vi "Teleop.vi"(10 "Match Info":T1={"Autonomous Elapsed Seconds"=0.0, "TeleOp Elapsed Seconds"=0.0, "Disabled Elapsed Seconds"=0.0, "Visited Autonomous"=FALSE, "Visited TeleOp"=FALSE, "Visited Disabled"=FALSE, "Autonomous Settings"={"Autonomous Style"=enum."Independent", "VI Refnum"=refnum}}, 11 "Call Context":T2) -> ()   [LabVIEW 2016]
doc: "This VI is called for each TeleOp packet received from the DS where the robot is not disabled. It is often used to read from the joysticks and update I/O or to update setpoints for timed control loops. It should complete and return within 20 milliseconds or it may miss DS packets."
uses:
  <vilib>/Rock Robotics/WPI/DriverStation/WPI_DriverStationDerivedRobotMode.ctl
  <vilib>/Rock Robotics/WPI/DriverStation/WPI_DriverStationMatch Info.ctl
  <vilib>/Rock Robotics/WPI/Utilities/WPI_GetSetVariantRefNum.vi
  <vilib>/Rock Robotics/Network Tables/NT Write Boolean.vi
  <vilib>/Rock Robotics/Network Tables/NT Write Boolean Array.vi
  <vilib>/Rock Robotics/Network Tables/NT Write Numeric Array.vi
  <vilib>/Rock Robotics/WPI/Solenoid/Deprecated/WPI_SolenoidSetBool.vi
  <vilib>/Rock Robotics/WPI/Ultrasonic/WPI_SonarMB1010AnalogRefNum Registry Get.vi
  <vilib>/Rock Robotics/WPI/Ultrasonic/WPI_SonarMB1010AnalogGetRange.vi
  <vilib>/Rock Robotics/Network Tables/NT Read Number.vi
  <vilib>/Rock Robotics/Network Tables/NT Write Number.vi
panel:
  out "gyro":dbl
  out "sonar distance (inches)":dbl
  out "Encoder Loop 2":string
  out "Encoder Loop":dbl
  out "Encoder Rate":dbl
  out "Encoder State":string
  out "Encoder Direction":string
  out "Distance 2":dbl
  out "Angle 2":dbl
  out "Distance":dbl
  out "Enabled":bool
  out "Compressor Running":bool
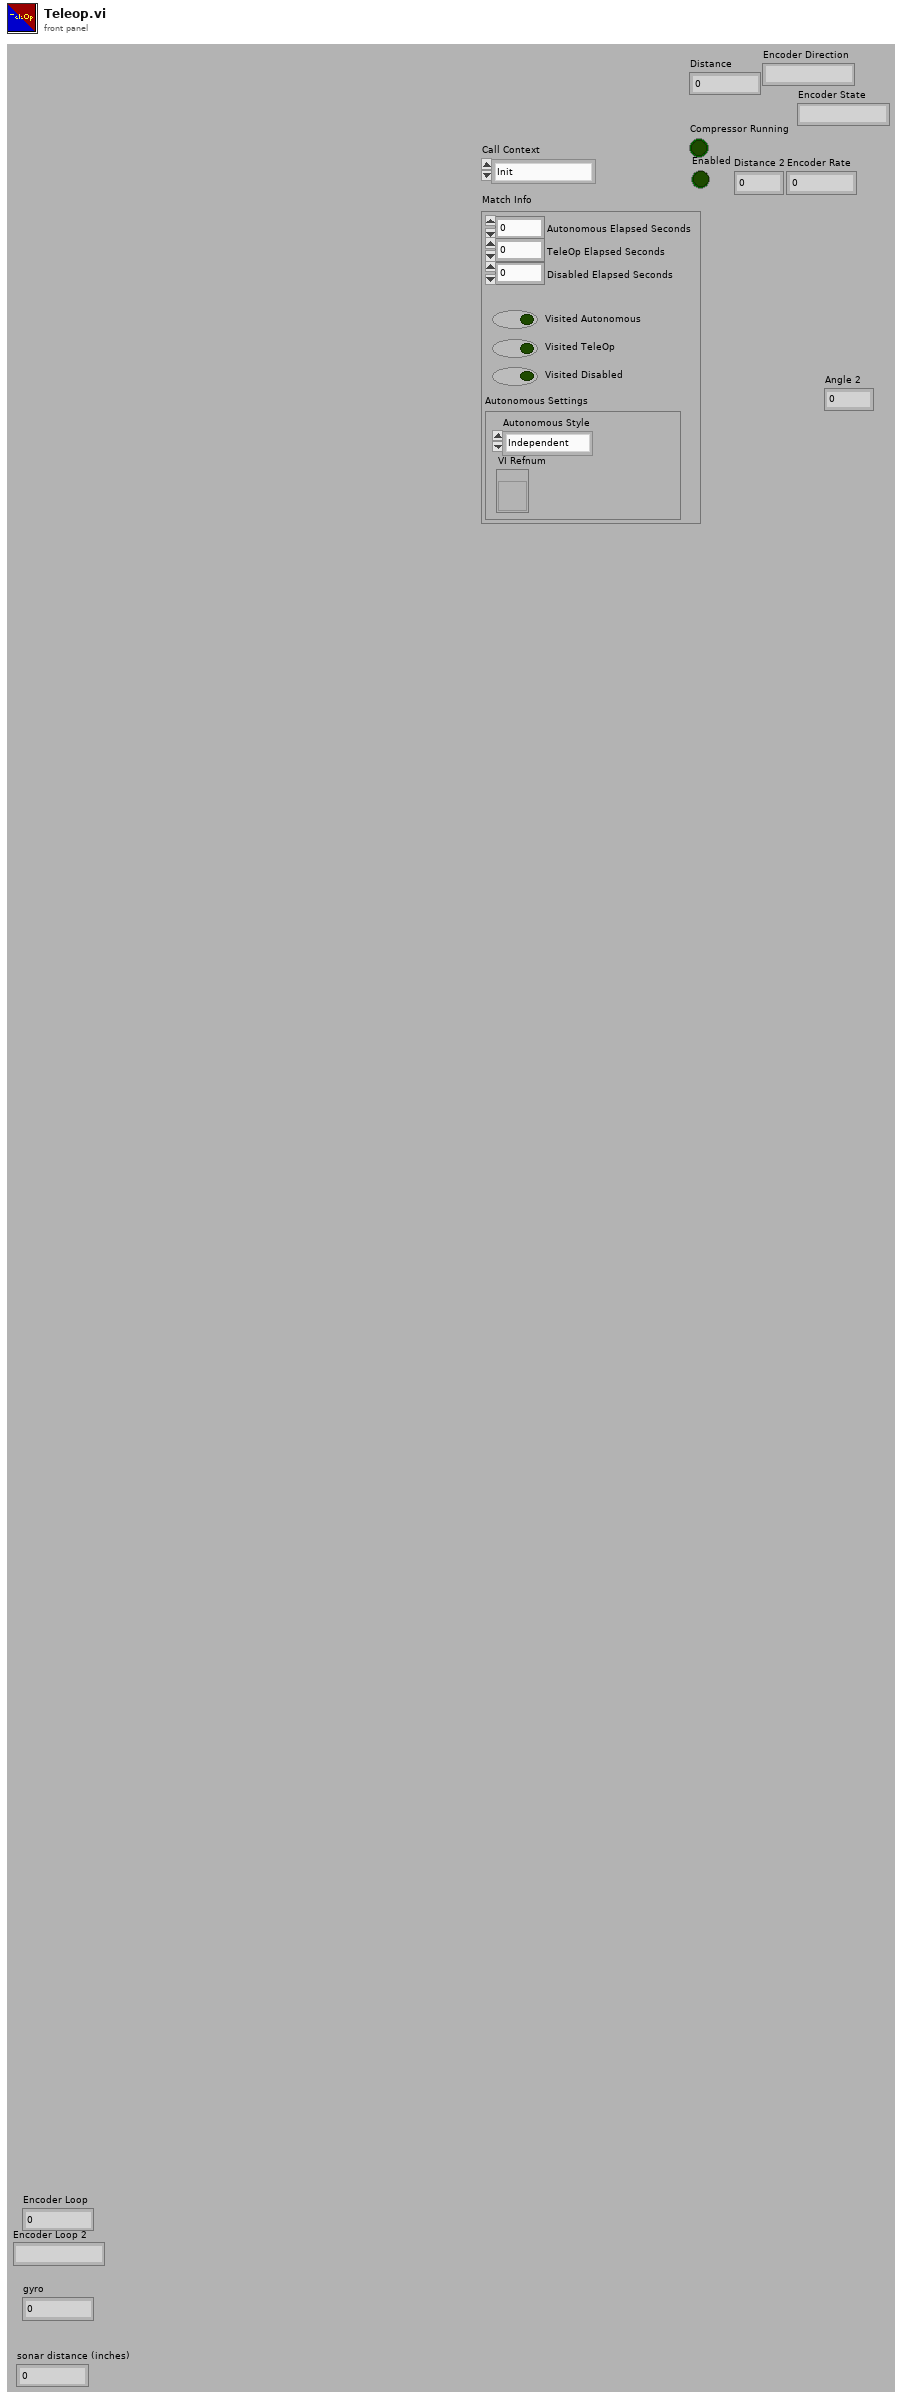
[diagram p1: front panel]
types:
  T1 = typedef "WPI_DriverStationMatch Info.ctl" = cluster{"Autonomous Elapsed Seconds":dbl, "TeleOp Elapsed Seconds":dbl, "Disabled Elapsed Seconds":dbl, "Visited Autonomous":bool, "Visited TeleOp":bool, "Visited Disabled":bool, "Autonomous Settings":cluster{"Autonomous Style":enum16{"Iterative", "Independent"}, "VI Refnum":refnum<vi>}}
  T2 = typedef "WPI_DriverStationDerivedRobotMode.ctl" = enum16{"Init", "Execute", "Stop"}
  T3 = typedef "WPI_EncoderDevRef.ctl" = cluster{"DevStatus":errorcluster, "EncoderIndex":T4, "CounterIndex":T5, "DistancePerCount":dbl, "Decoding Type":T6}
  T4 = typedef "FPGA_EncoderIdx.ctl" = enum8{"Enc 0", "Enc 1", "Enc 2", "Enc 3", "Enc 4", "Enc 5", "Enc 6", "Enc 7", "Invalid"}
  T5 = typedef "FPGA_CounterCtrSystemIndex.ctl" = enum8{"Ctr 0", "Ctr 1", "Ctr 2", "Ctr 3", "Ctr 4", "Ctr 5", "Ctr 6", "Ctr 7", "Invalid"}
  T6 = typedef "WPI_EncoderType.ctl" = enum16{"1x", "2x", "4x"}
  T7 = typedef "WPI_JoystickDevRef.ctl" = cluster{"Device":T8}
  T8 = typedef "WPI_JoystickDeviceEnum.ctl" = enum16{"USB 0", "USB 1", "USB 2", "USB 3", "USB 4", "USB 5"}
  T9 = typedef "WPI_GyroDevRef.ctl" = cluster{"DevStatus":errorcluster, "Analog Channel":T10, "Offset":dbl, "Gain (VoltsPerDegree/Second)":dbl, "Gyro Type":enum16{"Analog", "XRS450"}, "Handle":i32, "SPI Bus":T11, "Device Found":bool, "Sample Rate":dbl, "Calibrate On Open":bool}
  T10 = typedef "FPGA_AIChannel.ctl" = enum8{"AI 0", "AI 1", "AI 2", "AI 3", "AI MXP 0", "AI MXP 1", "AI MXP 2", "AI MXP 3", "Invalid"}
  T11 = typedef "spi_bus.ctl" = enum16{"SPI On-Board, CS0", "SPI On-Board, CS1", "SPI On-Board, CS2", "SPI On-Board, CS3", "SPI MXP", "Invalid"}
  T12 = typedef "WPI_CompressorDevRef.ctl" = cluster{"DevStatus":errorcluster, "Pneumatics Control Module":u8}
  T13 = typedef "WPI_SonarMB1010AnalogDeviceRef.ctl" = cluster{"AIDeviceRef":T14, "Scaling factor (V/in)":dbl, "Average Bits":u8}
  T14 = typedef "WPI_AnalogChannelDevRef.ctl" = cluster{"DevStatus":errorcluster, "Analog Channel":T10}
  T15 = typedef "WPI_SolenoidDevRef.ctl" = cluster{"DevStatus":errorcluster, "Pneumatics Control Module":u8, "Forward Solenoid Channel":T16, "Reverse Solenoid Channel":T16}
  T16 = typedef "WPI_SolenoidChannel.ctl" = enum8{"Solenoid 0", "Solenoid 1", "Solenoid 2", "Solenoid 3", "Solenoid 4", "Solenoid 5", "Solenoid 6", "Solenoid 7", "Invalid"}
  T17 = typedef "WPI_RobotDriveDevRef.ctl" = cluster{"DevStatus":errorcluster, "Motors[]":T18[], "Square Inputs":bool, "Max Output":dbl}
  T18 = typedef "WPI_MotorControlDeviceRef.ctl" = cluster{"DeviceStatus":errorcluster, "Type":T19, "PWM":cluster{"PWM Channel":T20, "DeadBand":T21}, "CAN":cluster{"Device Number":u8, "SetOutput VI Ref":variant, "GetOutput VI Ref":variant, "Enable VI Ref":variant, "Disable VI Ref":variant, "Data":variant}, "Invert":bool}
  T19 = typedef "WPI_MotorControlType.ctl" = enum16{"PWM", "CAN"}
  T20 = typedef "FPGA_DIOPWMChannel.ctl" = enum8{"PWM 0", "PWM 1", "PWM 2", "PWM 3", "PWM 4", "PWM 5", "PWM 6", "PWM 7", "PWM 8", "PWM 9", "PWM MXP 0", "PWM MXP 1", "PWM MXP 2", "PWM MXP 3", "PWM MXP 4", "PWM MXP 5", "PWM MXP 6", "PWM MXP 7", "PWM MXP 8", "PWM MXP 9", "Invalid"}
  T21 = typedef "WPI_PWMDeadband.ctl" = cluster{"Name":string, "maxPositivePwm":i32, "minPositivePwm":i32, "centerPwm":i32, "maxNegativePwm":i32, "minNegativePwm":i32, "angularRange":u16}
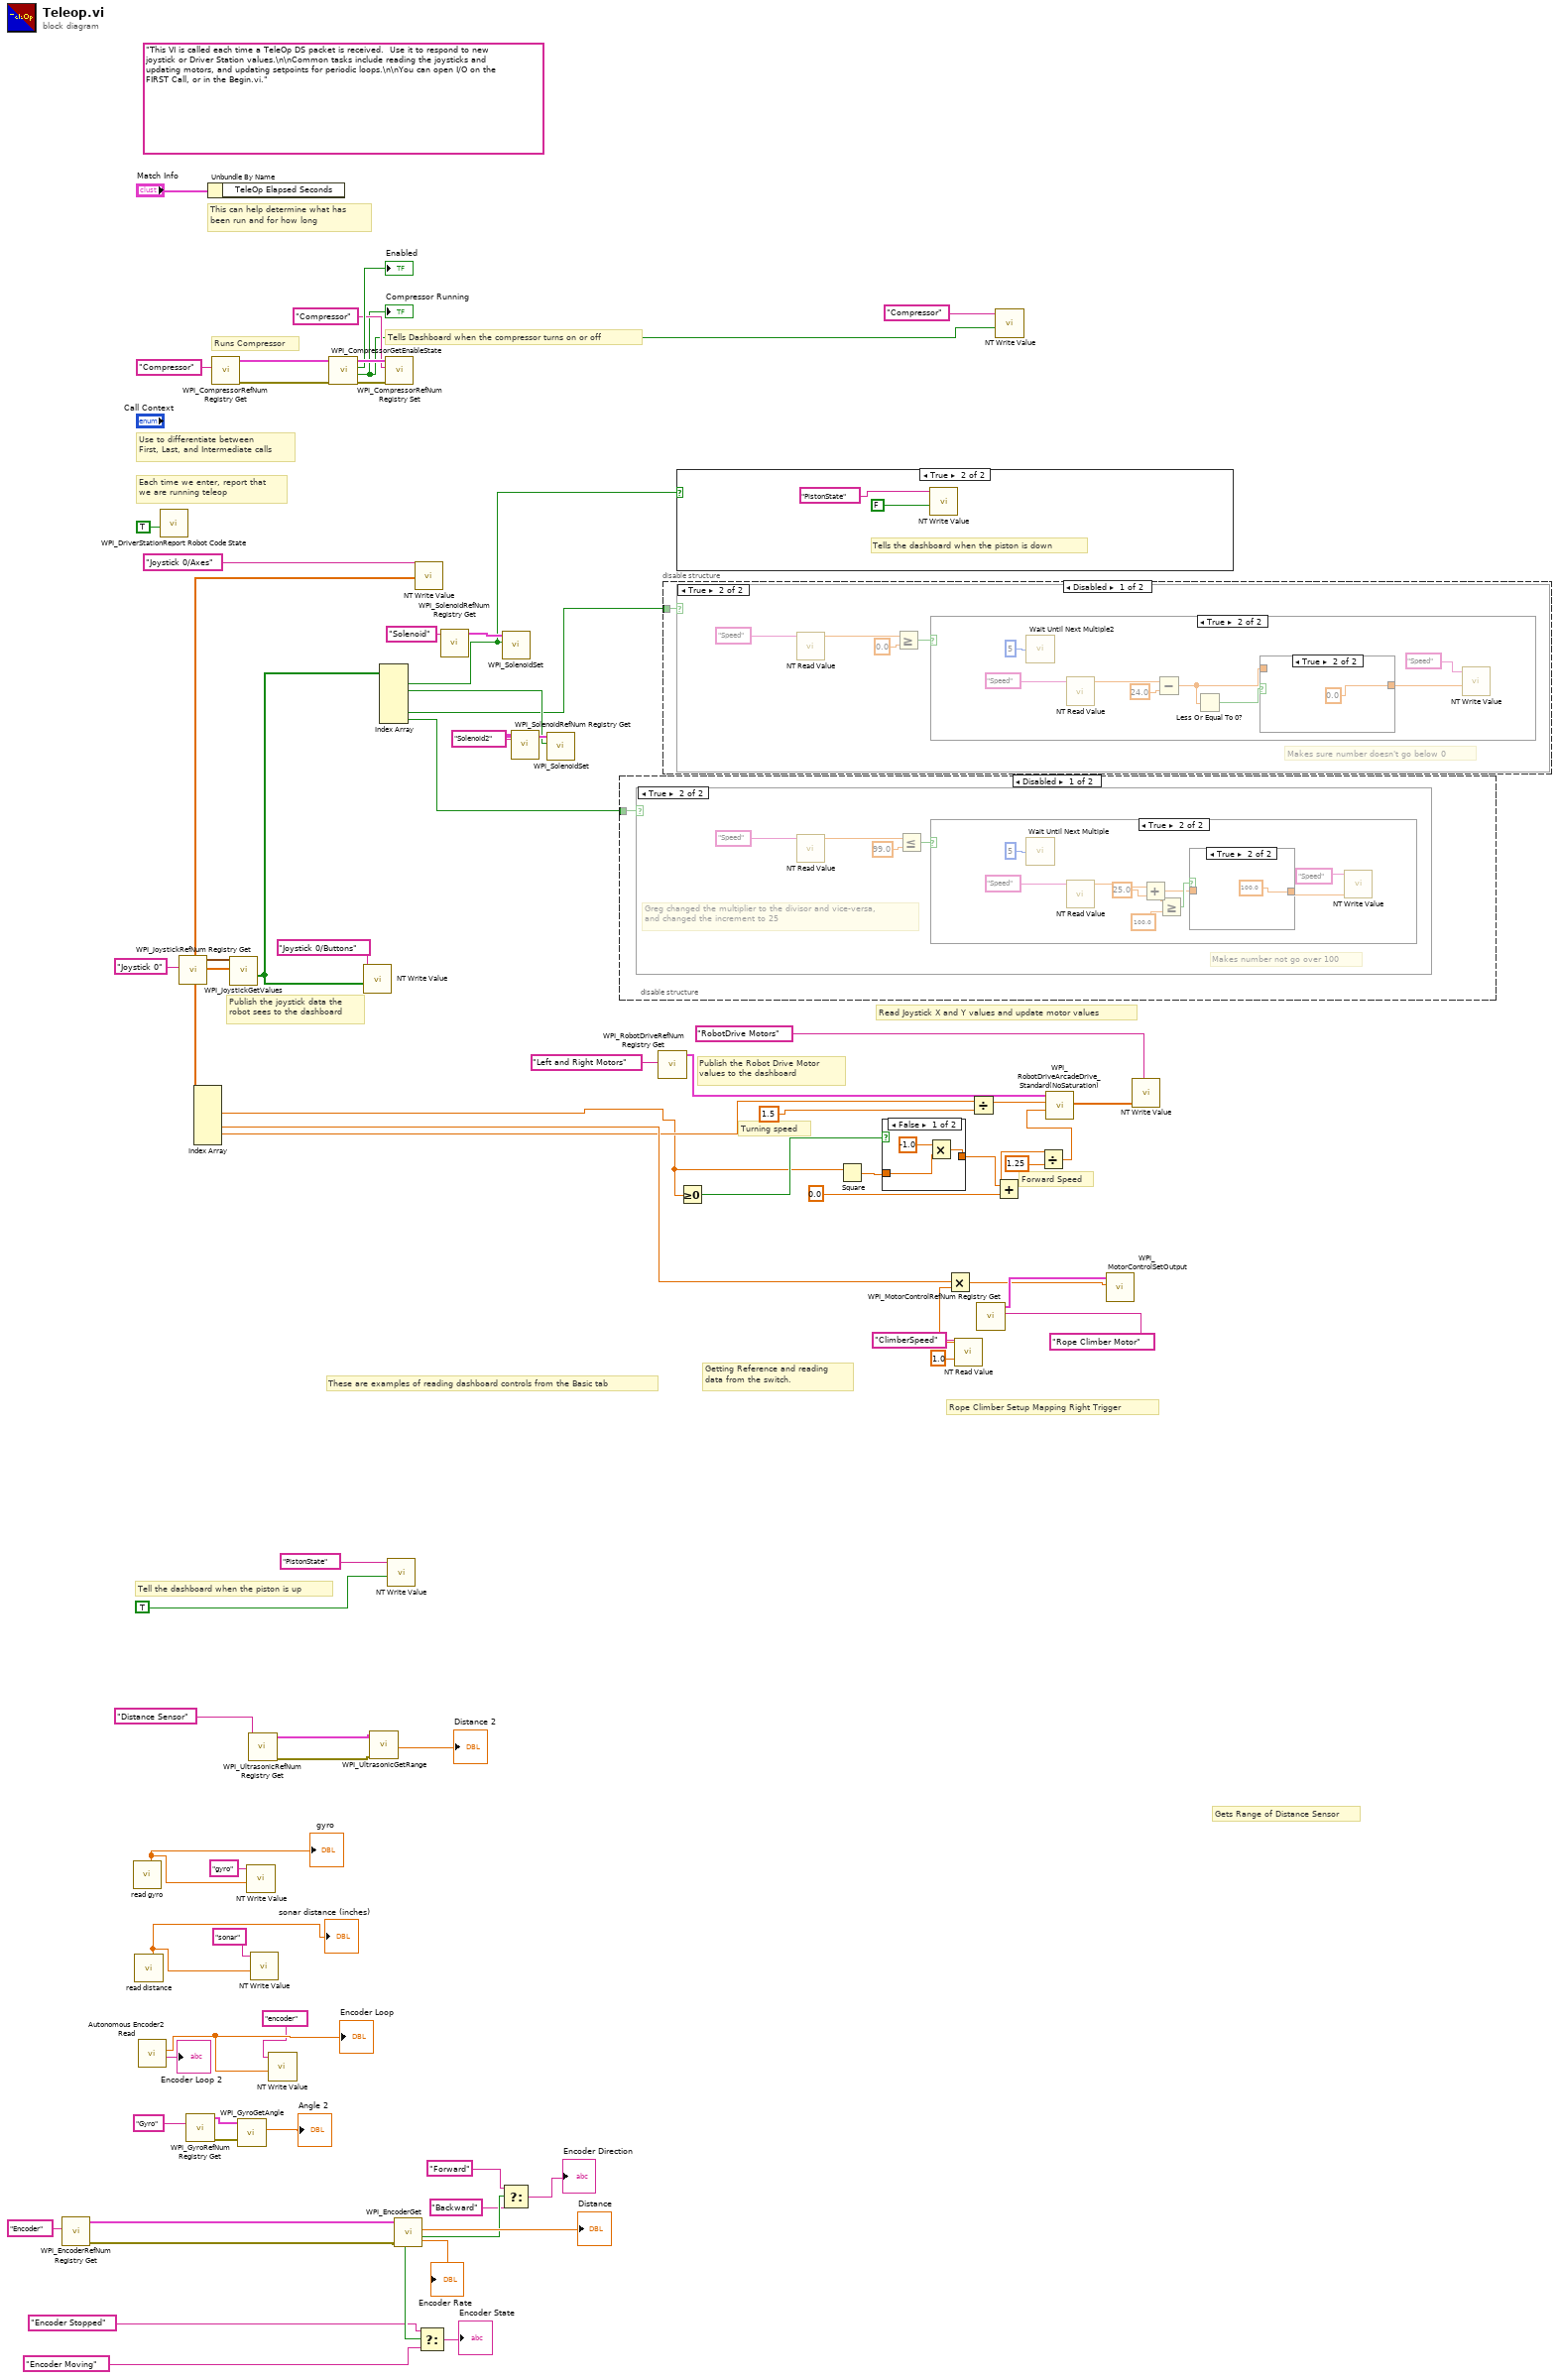
[diagram p0: block diagram]
diagram:
  (unwired) "This VI is called each time a TeleOp DS packet is received.  Use it to respond to new joystick or Driver Station values.\n\nCommon tasks include reading the joysticks and updating motors, and updating setpoints for periodic loops.\n\nYou can open I/O on the FIRST Call, or in the Begin.vi."
  # "Turning speed"
  # "Forward Speed"
  # "Rope Climber Setup Mapping Right Trigger"
  # "Gets Range of Distance Sensor"
  # "Getting Reference and reading \ndata from the switch."
  # "Tell the dashboard when the piston is up"
  # "Publish the joystick data the\nrobot sees to the dashboard"
  # "Publish the Robot Drive Motor\nvalues to the dashboard"
  # "Read Joystick X and Y values and update motor values"
  # "Tells Dashboard when the compressor turns on or off"
  # "Runs Compressor"
  # "These are examples of reading dashboard controls from the Basic tab"
  # "Each time we enter, report that\nwe are running teleop"
  # "Use to differentiate between\nFirst, Last, and Intermediate calls"
  # "This can help determine what has\nbeen run and for how long"
  n1 = call <vilib>:"WPI_EncoderRefNum Registry Get.vi"("refnum name"="Encoder") -> ("error out"=w41:errorcluster, "EncoderDevRef"=w42:T3)  [unwired: 9 in]
  n2 = call "read gyro.vi"() -> ("Angle 2"=w14:dbl)  [unwired: 10 in, 1 out]
  "gyro" <- w14
  n3 = call "read distance.vi"() -> ("Distance 2"=w12:dbl)  [unwired: 10 in, 1 out]
  "sonar distance (inches)" <- w12
  n4 = call "Autonomous Encoder2 Read.vi"() -> ("Encoder Direction"=→"Encoder Loop 2":string, "Encoder Distance"=w9:dbl)  [unwired: 9 in, 1 out]
  "Encoder Loop" <- w9
  n5 = call <vilib>:"WPI_DriverStationReport Robot Code State.vi"("TeleOp"=TRUE ("Autonomous")) -> ()  [unwired: 10 in, 1 out]
  n6 = call <vilib>:"WPI_JoystickRefNum Registry Get.vi"("refnum name"="Joystick 0") -> ("JoystickDevRef"=w63:T7)  [unwired: 1 in, 9 out]
  n7 = call <vilib>:"WPI_GyroRefNum Registry Get.vi"("refnum name"="Gyro") -> ("error out"=w36:errorcluster, "GyroDevRef"=w37:T9)  [unwired: 9 in]
  n8 = Unbundle By Name("Match Info") -> ()  [unwired: 1 out]
  n9 = call <vilib>:"WPI_CompressorRefNum Registry Get.vi"("refnum name"="Compressor") -> ("error out"=w73:errorcluster, "CompressorDevRef"=w75:T12)  [unwired: 9 in]
  n10 = call <vilib>:"WPI_JoystickGetValues.vi"("JoystickDevRef"=w63) -> ("Buttons"=w57:bool[], "Axes"=w60:dbl[])  [unwired: 6 in, 3 out]
  n11 = Index Array(array=w60) -> (element #2=w7:dbl, element #4=w46:dbl, element #5=w22:dbl)  [unwired: 6 in, 3 out]
  n12 = call <vilib>:"WPI_GyroGetAngle.vi"("error in"=w36, "GyroDevRef"=w37) -> ("Angle"=→"Angle 2":dbl)  [unwired: 5 in, 4 out]
  n13 = call-poly <vilib>:"NT Write Value.vi"("Numeric"=w14, "Name"="gyro") -> ()  [unwired: 9 in, 1 out]
  n14 = call-poly <vilib>:"WPI_UltrasonicRefNum Registry Get.vi"("refnum name"="Distance Sensor") -> ("error out"=w32:errorcluster, "SonarMB1010AnalogDevRef"=w34:T13)  [unwired: 9 in]
  n15 = call-poly <vilib>:"NT Write Value.vi"("Numeric"=w12, "Name"="sonar") -> ()  [unwired: 9 in, 1 out]
  n16 = call-poly <vilib>:"NT Write Value.vi"("Numeric"=w9, "Name"="encoder") -> ()  [unwired: 9 in, 1 out]
  n17 = call <vilib>:"WPI_CompressorGetEnableState.vi"("error in (no error)"=w73, "CompressorDevRef"=w75) -> ("error out"=w72:errorcluster, "Compressor Running"=w67:bool, "Enabled"=→"Enabled":bool, "CompressorDevRef"=w74:T12)  [unwired: 6 in]
  "Compressor Running" <- w67
  n18 = call-poly <vilib>:"NT Write Value.vi"("Boolean Array"=w57, "Name"="Joystick 0/Buttons") -> ()  [unwired: 9 in, 1 out]
  n19 = call-poly <vilib>:"WPI_UltrasonicGetRange.vi"("error in"=w32, "SonarMB1010AnalogDevRef"=w34) -> ("Distance"=→"Distance 2":dbl)  [unwired: 7 in, 2 out]
  n20 = Index Array(array=w57) -> (element #1=w51:bool, element #2=w52:bool, element #5=w47:bool, element #6=w48:bool)  [unwired: 6 in, 2 out]
  n21 = call <vilib>:"WPI_CompressorRefNum Registry Set.vi"("error in (no error)"=w72, "refnum name"="Compressor", "CompressorDevRef"=w74) -> ()  [unwired: 7 in, 2 out]
  n22 = call-poly <vilib>:"NT Write Value.vi"("Boolean"=TRUE, "Name"="PistonState") -> ()  [unwired: 9 in, 1 out]
  n23 = call <vilib>:"WPI_EncoderGet.vi"("error in (no error)"=w41, "EncoderDevRef"=w42) -> ("Direction"=w31:bool, "Distance"=→"Distance":dbl, "Rate"=→"Encoder Rate":dbl, "Stopped"=w27:bool)  [unwired: 4 in, 2 out]
  n24 = call-poly <vilib>:"NT Write Value.vi"("Numeric Array"=w60, "Name"="Joystick 0/Axes") -> ()  [unwired: 9 in, 1 out]
  n25 = Select(t="Encoder Stopped", s=w27, f="Encoder Moving") -> (s? t:f=→"Encoder State":string)
  n26 = call <vilib>:"WPI_SolenoidRefNum Registry Get.vi"("refnum name"="Solenoid") -> ("SolenoidDevRef"=w53:T15)  [unwired: 9 in, 1 out]
  n27 = call-poly <vilib>:"WPI_SolenoidSet.vi"("Value"=w51, "SolenoidDevRef"=w53) -> ()  [unwired: 8 in, 2 out]
  n28 = Select(t="Forward", s=w31, f="Backward") -> (s? t:f=→"Encoder Direction":string)
  n29 = call <vilib>:"WPI_SolenoidRefNum Registry Get.vi"("refnum name"="Solenoid2") -> ("SolenoidDevRef"=w55:T15)  [unwired: 9 in, 1 out]
  n30 = call-poly <vilib>:"WPI_SolenoidSet.vi"("Value"=w52, "SolenoidDevRef"=w55) -> ()  [unwired: 8 in, 2 out]
  n31 = disable-structure shown="Disabled" {
    disable-tunnel: w48 -> [w78 _]
    frame Disabled {
      n32 = case shown="True" w78 {
        frame False {
        }
        frame True {
          # "Makes number not go over 100"
          # "Greg changed the multiplier to the divisor and vice-versa,\nand changed the increment to 25"
          n33 = call-poly <vilib>:"NT Read Value.vi"("Name"="Speed") -> ("Numeric"=w80:dbl)  [unwired: 9 in, 1 out]
          n34 = Less Or Equal?(x=w80, y=99.0) -> (x <= y?=w81:bool)
          n35 = case shown="True" w81 {
            frame False {
            }
            frame True {
              n36 = call "Wait Until Next Multiple"("Count(mSec)"=u32 5) -> ()  [unwired: 1 out]
              n37 = call-poly <vilib>:"NT Read Value.vi"("Name"="Speed") -> ("Numeric"=w88:dbl)  [unwired: 9 in, 1 out]
              n38 = Add(x=w88, y=25.0) -> (x+y=w83:dbl)
              n39 = Greater Or Equal?(x=w83, y=100.0) -> (x >= y?=w85:bool)
              n40 = case shown="True" w85 {
                tunnel: [w92 100.0 ("Numeric")] -> w86
                tunnel: w83 -> [w92 _]
                frame False {
                }
                frame True {
                }
              }
              n41 = call-poly <vilib>:"NT Write Value.vi"("Numeric"=w86, "Name"="Speed") -> ()  [unwired: 9 in, 1 out]
            }
          }
        }
      }
    }
    frame Enabled {
    }
  }
  n42 = call <vilib>:"WPI_RobotDriveRefNum Registry Get.vi"("refnum name"="Left and Right Motors") -> ("RobotDriveDevRef"=w65:T17)  [unwired: 1 in, 9 out]
  n43 = disable-structure shown="Disabled" {
    disable-tunnel: w47 -> [w94 _]
    frame Disabled {
      n44 = case shown="True" w94 {
        frame False {
        }
        frame True {
          # "Makes sure number doesn't go below 0"
          n45 = call-poly <vilib>:"NT Read Value.vi"("Name"="Speed") -> ("Numeric"=w97:dbl)  [unwired: 9 in, 1 out]
          n46 = Greater Or Equal?(x=w97, y=0.0) -> (x >= y?=w95:bool)
          n47 = case shown="True" w95 {
            frame False {
            }
            frame True {
              n48 = call "Wait Until Next Multiple2"("Count(mSec)"=u32 5) -> ()  [unwired: 1 out]
              n49 = call-poly <vilib>:"NT Read Value.vi"("Name"="Speed") -> ("Numeric"=w105:dbl)  [unwired: 9 in, 1 out]
              n50 = Subtract(x=w105, y=24.0) -> (x-y=w99:dbl)
              n51 = Less Or Equal To 0?(x=w99) -> (x <= 0?=w101:bool)
              n52 = case shown="True" w101 {
                tunnel: [w107 0.0 ("Numeric")] -> w100
                tunnel: w99 -> [w107 _]
                frame False {
                }
                frame True {
                }
              }
              n53 = call-poly <vilib>:"NT Write Value.vi"("Numeric"=w100, "Name"="Speed") -> ()  [unwired: 9 in, 1 out]
            }
          }
        }
      }
    }
    frame Enabled {
    }
  }
  n54 = case shown="True" w51 {
    frame False {
    }
    frame True {
      # "Tells the dashboard when the piston is down"
      n55 = call-poly <vilib>:"NT Write Value.vi"("Boolean"=FALSE, "Name"="PistonState") -> ()  [unwired: 9 in, 1 out]
    }
  }
  n56 = Greater Or Equal To 0?(x=w7) -> (x >= 0?=w17:bool)
  n57 = Square(x=w7) -> (x^2=w16:dbl)
  n58 = case shown="False" w17 {
    tunnel: w16 -> [w113 w114]
    tunnel: [w111 w114] -> w15
    frame False {
      n59 = Multiply(x=-1.0, y=w113) -> (x*y=w111:dbl)
    }
    frame True {
    }
  }
  n60 = call-poly <vilib>:"NT Read Value.vi"("Default Value"=1.0, "Name"="ClimberSpeed") -> ("Numeric"=w3:dbl)  [unwired: 8 in, 1 out]
  n61 = Multiply(x=w46, y=w3) -> (x*y=w2:dbl)
  n62 = Divide(x=w22, y=1.5) -> (x/y=w44:dbl)
  n63 = call <vilib>:"WPI_MotorControlRefNum Registry Get.vi"("refnum name"="Rope Climber Motor") -> ("MotorControlDevRef"=w5:T18)  [unwired: 9 in, 1 out]
  n64 = Add(x=w15, y=0.0) -> (x+y=w19:dbl)
  n65 = call-poly <vilib>:"NT Write Value.vi"("Boolean"=w67, "Name"="Compressor") -> ()  [unwired: 9 in, 1 out]
  n66 = Divide(x=w19, y=1.25) -> (x/y=w18:dbl)
  n67 = call <vilib>:"WPI_RobotDriveArcadeDrive_Standard(NoSaturation).vi"("Y axis value"=w18, "X axis value"=w44, "RobotDriveDevRef"=w65) -> ("Motor Values"=w59:dbl[])  [unwired: 1 in, 7 out]
  n68 = call <vilib>:"WPI_MotorControlSetOutput.vi"("Output"=w2, "MotorControlDevRef"=w5) -> ()  [unwired: 7 in, 3 out]
  n69 = call-poly <vilib>:"NT Write Value.vi"("Numeric Array"=w59, "Name"="RobotDrive Motors") -> ()  [unwired: 9 in, 1 out]
